vi "ZSliceCompute.vi"(9 "Function":T1, 11 "ZStack (um)":cluster{"Zstart":dbl, "Zstop":dbl, "Zstep":dbl}) -> (1 "# of Z-planes":i32, 2 "AOL Z Planes(um)":dbl[](array[numeric]) format="%#_12f", 3 "Motor Z Planes(um)":dbl[](array[numeric]) format="%#_12f", 5 "ZStack (um)":cluster{"Zstart":dbl, "Zstop":dbl, "Zstep":dbl})   [LabVIEW 2013]
uses:
  Typedefs/Read Write Enum.ctl
panel:
  # "SUBROUTINE"
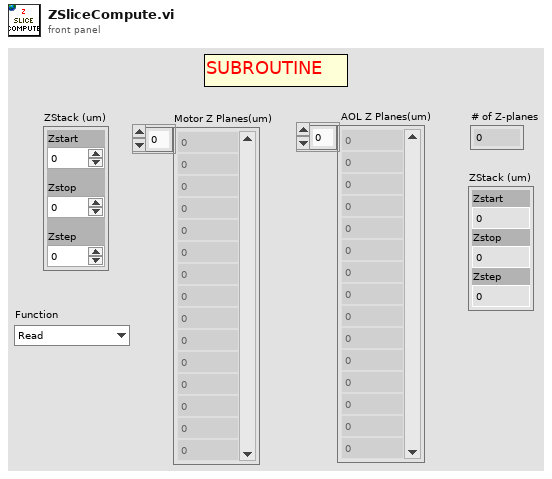
[diagram p1: front panel]
types:
  T1 = typedef "Read Write Enum.ctl" = enum16{"Read", "Write"}
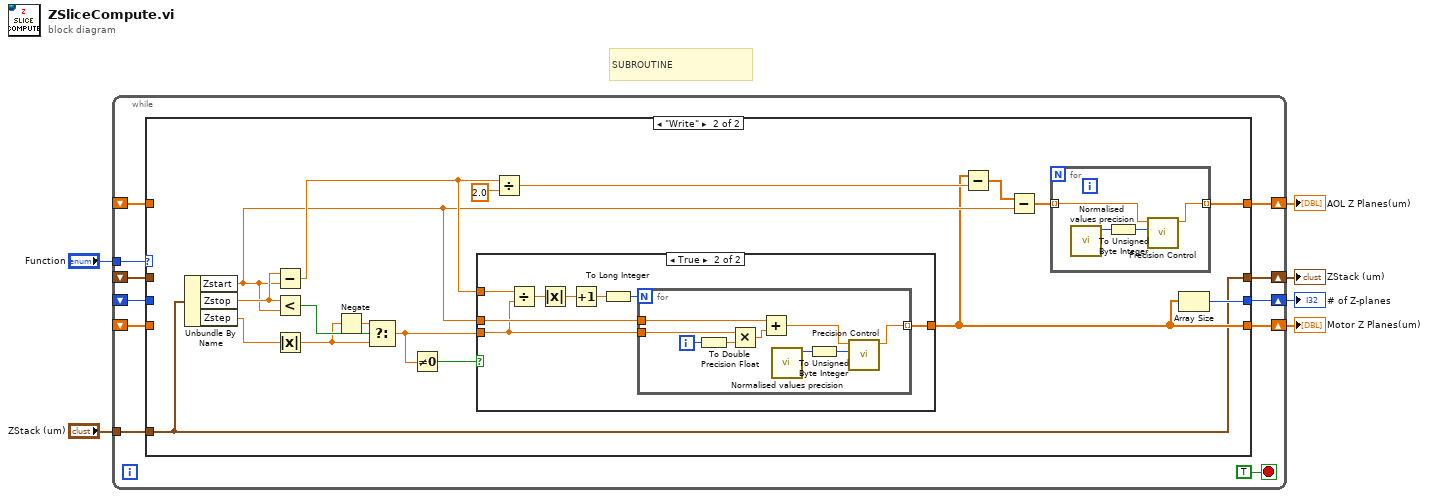
[diagram p0: block diagram]
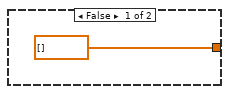
[diagram p3: hidden frame]
diagram:
  # "SUBROUTINE"
  n1 = while {
    shift-right: [w15] -> w5
    shift-left: _ -> [w10]
    shift-right: [w16] -> w6
    shift-left: _ -> [w11]
    shift-right: [w14] -> w4
    shift-left: _ -> [w12]
    tunnel: "Function" -> [w9]
    shift-right: [w8] -> w1
    shift-left: _ -> [w17]
    tunnel: "ZStack (um)" -> [w7]
    stop <- TRUE stop-if-true
    n2 = case shown="\"Write\"" w9 {
      tunnel: w17 -> [w18 _]
      tunnel: [w20 w26] -> w16
      tunnel: [w19 w25] -> w15
      tunnel: [w21 w23] -> w14
      tunnel: w12 -> [w21 _]
      tunnel: w11 -> [w20 _]
      tunnel: w10 -> [w19 _]
      tunnel: [w18 w22] -> w8
      tunnel: w7 -> [_ w22]
      frame "Read", Default {
      }
      frame "Write" {
        n3 = Unbundle By Name(w22) -> ("Zstart"=w27:dbl, "Zstop"=w35:dbl, "Zstep"=w34:dbl)
        n4 = Subtract(x=w35, y=w27) -> (x-y=w31:dbl)
        n5 = Less?(x=w35, y=w27) -> (x < y?=w38:bool)
        n6 = Absolute Value(x=w34) -> (abs(x)=w36:dbl)
        n7 = Negate(x=w36) -> (-x=w37:dbl)
        n8 = Select(t=w37, s=w38, f=w36) -> (s? t:f=w33:dbl)
        n9 = Not Equal To 0?(x=w33) -> (x != 0?=w32:bool)
        n10 = case shown="True" w32 {
          tunnel: w31 -> [_ w51]
          tunnel: w27 -> [_ w47]
          tunnel: w33 -> [_ w46]
          tunnel: [dbl[] [] w45] -> w25
          frame False {
          }
          frame True {
            n11 = Divide(x=w51, y=w46) -> (x/y=w48:dbl)
            n12 = Absolute Value(x=w48) -> (abs(x)=w49:dbl)
            n13 = Increment(x=w49) -> (x+1=w50:dbl)
            n14 = To Long Integer(number=w50) -> (32bit integer=w44:i32)
            n15 = for {
              N: w44 -> [_]
              tunnel: w46 -> [w59]
              tunnel: w47 -> [w58]
              tunnel: [w52] -> w45 mode=indexing
              i -> [w60]
              n16 = To Double Precision Float(number=w60) -> (double precision float=w56:dbl)
              n17 = Multiply(x=w59, y=w56) -> (x*y=w57:dbl)
              n18 = Add(x=w58, y=w57) -> (x+y=w53:dbl)
              n19 = call "Normalised values precision.vi"() -> ("Normalised values precision"=w54:i32)  [unwired: 11 in]
              n20 = To Unsigned Byte Integer(number=w54) -> (unsigned 8bit integer=w55:u8)
              n21 = call "Precision Control.vi"("Precision"=w55, "Input Value"=w53) -> ("Output Value"=w52:dbl)  [unwired: 8 in, 1 out]
            }
          }
        }
        n22 = Divide(x=w31, y=2.0) -> (x/y=w28:dbl)
        n23 = Subtract(x=w25, y=w28) -> (x-y=w29:dbl[])
        n24 = Subtract(x=w29, y=w27) -> (x-y=w24:dbl[])
        n25 = for {
          tunnel: [w40] -> w23 mode=indexing
          tunnel: w24 -> [w39] mode=indexing
          n26 = call "Normalised values precision.vi"() -> ("Normalised values precision"=w41:i32)  [unwired: 11 in]
          n27 = To Unsigned Byte Integer(number=w41) -> (unsigned 8bit integer=w42:u8)
          n28 = call "Precision Control.vi"("Precision"=w42, "Input Value"=w39) -> ("Output Value"=w40:dbl)  [unwired: 8 in, 1 out]
        }
        n29 = Array Size(array=w25) -> (size(s)=w26:i32)
      }
    }
  }
  "Motor Z Planes(um)" <- w5
  "AOL Z Planes(um)" <- w4
  "# of Z-planes" <- w6
  "ZStack (um)" <- w1
